vi "Process Repeats.vi"(11 "Control State in":refnum<class "Control State.lvclass">) -> (3 "Control State out":refnum<class "Control State.lvclass">)   [LabVIEW 2021, in "Control State.lvclass"]
uses:
  Control State.lvclass
  Control State.lvclass/Control State.ctl
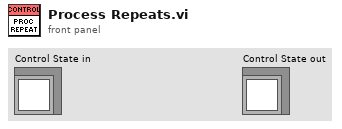
[diagram p1: front panel]
types:
  T1 = typedef "Control State.lvclass/Button State.ctl" = enum16{"Undefined", "Pressed", "Released", "Held", "Not Held"}
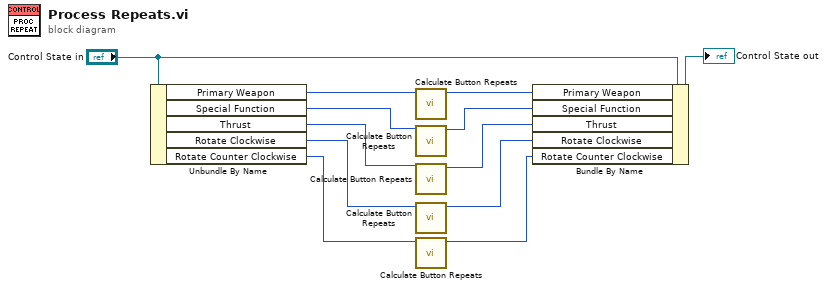
[diagram p0: block diagram]
diagram:
  n1 = Unbundle By Name("Control State in") -> ("Primary Weapon"=w10:T1, "Special Function"=w8:T1, "Thrust"=w6:T1, "Rotate Clockwise"=w4:T1, "Rotate Counter Clockwise"=w2:T1)
  n2 = call "Calculate Button Repeats.vi"("Previous Button State"=w10) -> ("New Buton State"=w9:T1)  [unwired: 10 in]
  n3 = call "Calculate Button Repeats.vi"("Previous Button State"=w8) -> ("New Buton State"=w7:T1)  [unwired: 10 in]
  n4 = call "Calculate Button Repeats.vi"("Previous Button State"=w6) -> ("New Buton State"=w5:T1)  [unwired: 10 in]
  n5 = call "Calculate Button Repeats.vi"("Previous Button State"=w4) -> ("New Buton State"=w3:T1)  [unwired: 10 in]
  n6 = call "Calculate Button Repeats.vi"("Previous Button State"=w2) -> ("New Buton State"=w1:T1)  [unwired: 10 in]
  n7 = Bundle By Name(cluster="Control State in", "Primary Weapon"=w9, "Special Function"=w7, "Thrust"=w5, "Rotate Clockwise"=w3, "Rotate Counter Clockwise"=w1) -> (→"Control State out":refnum<class "Control State.lvclass">)
